vi "DSF.Shared.Configuration.Transfer.Errors.Channels Not Contiguous.vi"(8 "error in (no error)":errorcluster, 10 "bad descriptor index":i32, 11 "Transfer Configuration in":refnum<class "DSF.Shared.Configuration.Transfer.lvclass">) -> (0 "error out":errorcluster, 3 "Transfer Configuration out":refnum<class "DSF.Shared.Configuration.Transfer.lvclass">)   [LabVIEW 2017, in "DSF.Shared.lvlib" / "DSF.Shared.Configuration.Transfer.lvclass"]
uses:
  DSF.Shared.Configuration.Transfer.lvclass
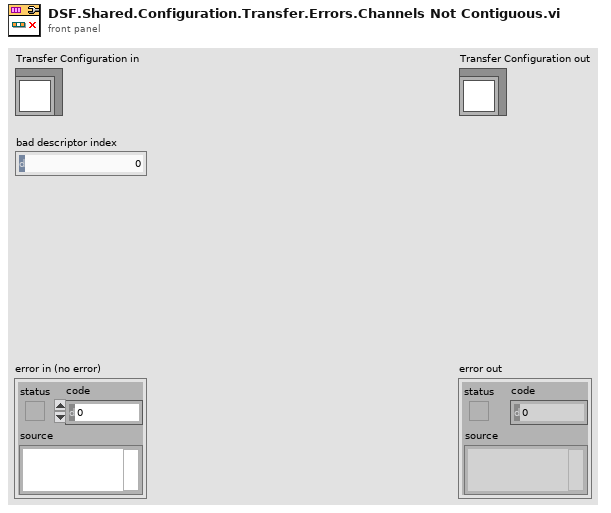
[diagram p1: front panel]
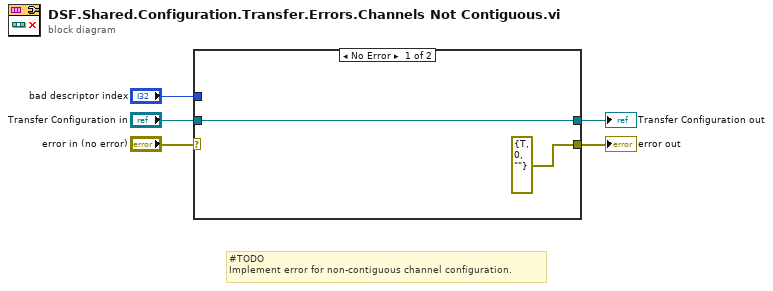
[diagram p0: block diagram]
diagram:
  # "#TODO\nImplement error for non-contiguous channel configuration."
  n1 = case shown="No Error" "error in (no error)" {
    selector: "error in (no error)" -> [_ w8]
    tunnel: [errorcluster {"status"=TRUE, "code"=0, "source"=""} ("error IO") w8] -> w4
    tunnel: "Transfer Configuration in" -> [w7 w9]
    tunnel: [w7 w9] -> w2
    tunnel: "bad descriptor index" -> [_ _]
    frame No Error {
    }
    frame Error {
    }
  }
  "error out" <- w4
  "Transfer Configuration out" <- w2
